vi "demod_fm_2.vi"(10 "Q input":u8, 11 "I input":u8) -> (3 "sample out":sgl)   [LabVIEW 2011]
doc: "Ez a VI végzi az FM demodulációt. A képlet: s=(I*dQ/dt - Q*dI/dt)/(I^2 + Q^2) A képlet származási helye: http://www.dsprelated.com/showmessage/142012/1.php"
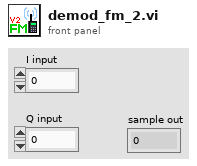
[diagram p1: front panel]
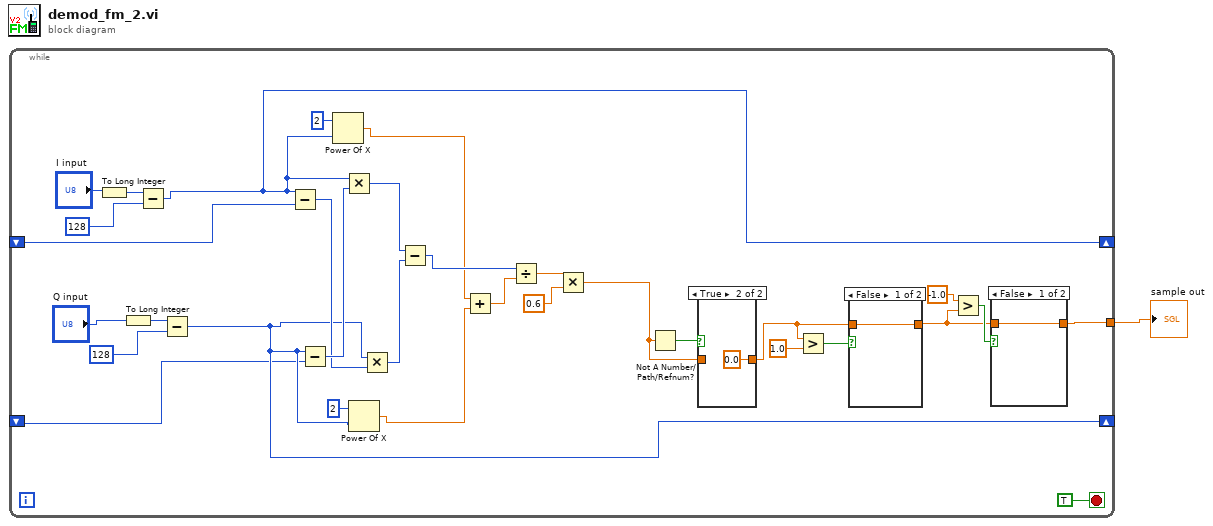
[diagram p0: block diagram]
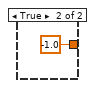
[diagram p2: hidden frame]
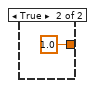
[diagram p3: hidden frame]
diagram:
  n1 = while {
    shift-right: [w15] -> _
    shift-left: _ -> [w13]
    shift-right: [w14] -> _
    shift-left: _ -> [w12]
    tunnel: [w2] -> w1
    stop <- TRUE stop-if-true
    n2 = To Long Integer(number="I input") -> (32bit integer=w26:i32)
    n3 = To Long Integer(number="Q input") -> (32bit integer=w23:i32)
    n4 = Subtract(x=w26, y=128) -> (x-y=w15:i32)
    n5 = Subtract(x=w23, y=128) -> (x-y=w14:i32)
    n6 = Subtract(x=w15, y=w13) -> (x-y=w31:i32)
    n7 = Subtract(x=w14, y=w12) -> (x-y=w32:i32)
    n8 = Power Of X(1:w15, 2:2 ("y")) -> (0:w21:dbl)
    n9 = Multiply(x=w15, y=w32) -> (x*y=w30:i32)
    n10 = Power Of X(1:w14, 2:2 ("y")) -> (0:w18:dbl)
    n11 = Multiply(x=w14, y=w31) -> (x*y=w29:i32)
    n12 = Subtract(x=w30, y=w29) -> (x-y=w28:i32)
    n13 = Add(x=w21, y=w18) -> (x+y=w27:dbl)
    n14 = Divide(x=w28, y=w27) -> (x/y=w11:dbl)
    n15 = Multiply(x=w11, y=0.6) -> (x*y=w4:dbl)
    n16 = Not A Number/Path/Refnum?(number/path/refnum=w4) -> (NaN/Path/Refnum?=w17:bool)
    n17 = case shown="True" w17 {
      tunnel: [w38 0.0] -> w3
      tunnel: w4 -> [w38 _]
      frame False {
      }
      frame True {
      }
    }
    n18 = Greater?(x=w3, y=1.0) -> (0:w9:bool)
    n19 = case shown="False" w9 {
      tunnel: w3 -> [w36 _]
      tunnel: [w36 1.0] -> w5
      frame False {
      }
      frame True {
      }
    }
    n20 = Greater?(x=-1.0 ("y"), y=w5) -> (0:w7:bool)
    n21 = case shown="False" w7 {
      tunnel: w5 -> [w34 _]
      tunnel: [w34 -1.0] -> w2
      frame False {
      }
      frame True {
      }
    }
  }
  "sample out" <- w1
